vi "IO.Create.vi"(8 "error in (no error)":errorcluster, 10 "IO Control":T2 {"Signals"."Response"."Byte Order" items=["Little Endian", "Big Endian"]; "Signals"."Response"."Data Type" items=["Signed", "Unsigned", "IEEE Float"]; "Signals"."Cmd"."Byte Order" items=["Little Endian", "Big Endian"]; "Signals"."Cmd"."Data Type" items=["Signed", "Unsigned", "IEEE Float"]}, 11 "Section Ptr":T1 format="%.0x") -> (0 "error out":errorcluster, 3 "Parent Ref out":T1 format="%.0x")   [LabVIEW 2015, in "Diagnostics Addon System Explorer.lvlib"]
uses:
  Diagnostics Addon System Explorer.lvlib
  Types/IO.Export.ctl
  Types/CmdResp.Export.ctl
  Shared/Types/Signal.ctl
  <vilib>/NI Veristand/Custom Device API/Custom Device Item Ref.ctl
  Types/FG.Action.ctl
  Shared/Types/Type.ctl
  <vilib>/NI Veristand/Custom Device API/NI VeriStand - Get Item Property.vi
  <vilib>/NI Veristand/Custom Device API/Get Item Property (U32).vi
  <vilib>/NI/NI VeriStand SysDef Utilities/SysDef API/SysDef.Property.Set.vi
  <vilib>/NI/NI VeriStand SysDef Utilities/_SubVIs/SysDef.Property.Set.U32.vi
  Shared/SubVIs/Constants.vi
  Shared/Diagnostics Addon Shared.lvlib
  <vilib>/NI/NI VeriStand SysDef Utilities/System Definition Utilities.lvlib
  <vilib>/NI VeriStand/Custom Device API/Custom Device API.lvlib
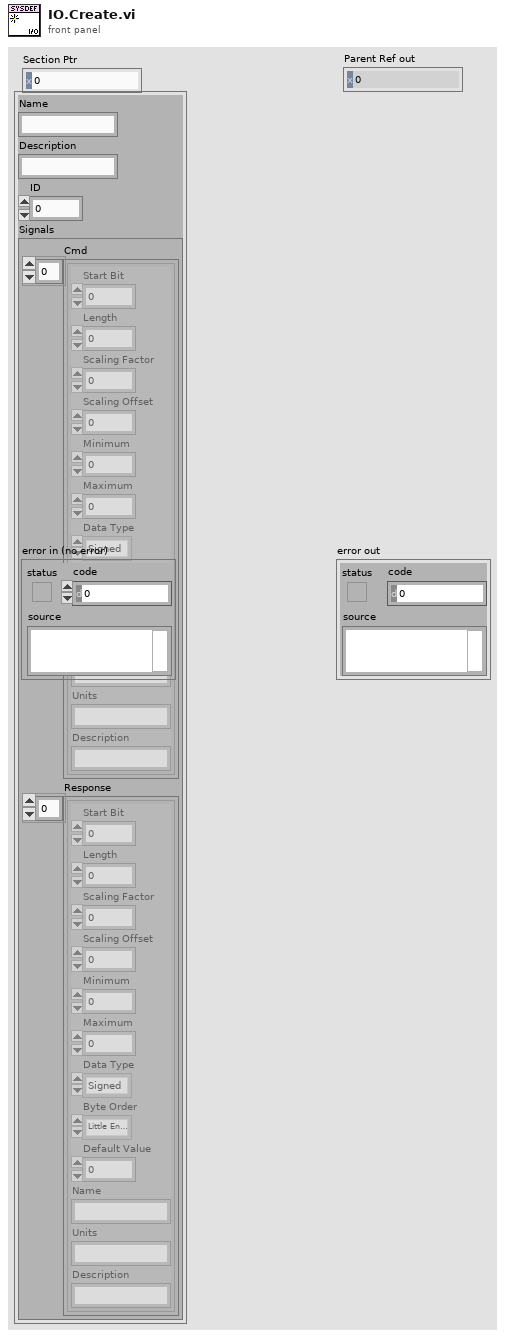
[diagram p1: front panel]
types:
  T1 = typedef "Custom Device API.lvlib/Custom Device Item Ref.ctl" = u64
  T2 = typedef "Diagnostics Addon System Explorer.lvlib/IO.Export.ctl" = cluster{"Name":string, "Description":string, "ID":u16, "Signals":T3}
  T3 = typedef "Diagnostics Addon System Explorer.lvlib/CmdResp.Export.ctl" = cluster{"Cmd":T4[], "Response":T4[]}
  T4 = typedef "Diagnostics Addon Shared.lvlib/Signal.ctl" = cluster{"Start Bit":u32, "Length":u32, "Scaling Factor":dbl, "Scaling Offset":dbl, "Minimum":dbl, "Maximum":dbl, "Data Type":u32, "Byte Order":u32, "Default Value":dbl, "Name":string, "Units":string, "Description":string}
  T5 = typedef "Diagnostics Addon Shared.lvlib/Type.ctl" = enum16{"DID", "CDID", "PID", "CPID", "Read Memory", "Write Memory", "DTC Control", "IO Cmd", "IO Resp", "Routine Start Cmd", "Routine Start Resp", "Routine Request Cmd", "Routine Request Resp", "Routine Stop Cmd", "Routine Stop Resp", "UserDefined Cmd", "UserDefined Rsp"}
  T6 = typedef "Diagnostics Addon System Explorer.lvlib/FG.Action.ctl" = enum16{"Get", "Set"}
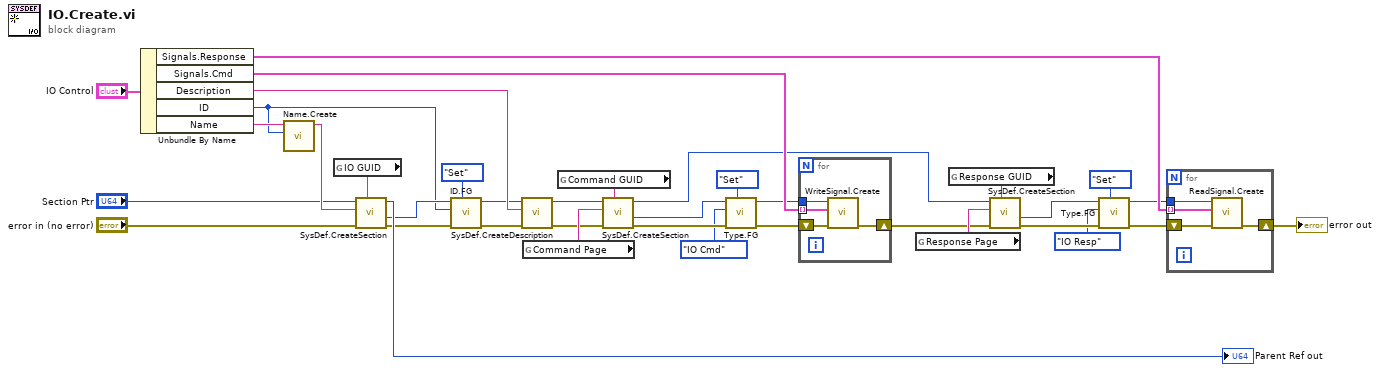
[diagram p0: block diagram]
diagram:
  n1 = Unbundle By Name("IO Control") -> ("Signals.Response"=w28:T4[], "Signals.Cmd"=w36:T4[], "Description"=w31:string, "ID"=w15:u16, "Name"=w18:string)
  n2 = call "Name.Create.vi"("PID Number"=w15, "PID Name"=w18) -> ("VS Name"=w37:string)  [unwired: 9 in]
  n3 = global read "Constants.vi" "IO GUID"() -> (w34:string)
  n4 = call <vilib>:"SysDef.CreateSection.vi"("GUID"=w34, "error in (no error)"="error in (no error)", "Name"=w37, "nodeID"="Section Ptr") -> ("error out"=w17:errorcluster, "New NodeID"=w16:u64, "nodeID out"=→"Parent Ref out":u64)  [unwired: 4 in, 1 out]
  n5 = call "ID.FG.vi"("Action"=FG.Action."Set", "error in (no error)"=w17, "ID"=w15, "Device Item Ref in"=w16) -> ("error out"=w13:errorcluster, "Device Item Ref out"=w12:T1)  [unwired: 5 in, 1 out]
  n6 = call <vilib>:"SysDef.CreateDescription.vi"("error in (no error)"=w13, "Description"=w31, "ID in"=w12) -> ("error out"=w22:errorcluster, "ID out"=w21:T1)  [unwired: 7 in]
  n7 = global read "Constants.vi" "Command Page"() -> (w27:string)
  n8 = global read "Constants.vi" "Command GUID"() -> (w26:string)
  n9 = call <vilib>:"SysDef.CreateSection.vi"("GUID"=w26, "error in (no error)"=w22, "Name"=w27, "nodeID"=w21) -> ("error out"=w10:errorcluster, "New NodeID"=w19:u64, "nodeID out"=w23:u64)  [unwired: 4 in, 1 out]
  n10 = call "Type.FG.vi"("Action"=FG.Action."Set", "error in (no error)"=w10, "Type"=Type."IO Cmd", "Device Item Ref in"=w19) -> ("error out"=w9:errorcluster, "Device Item Ref out"=w11:T1)  [unwired: 5 in, 1 out]
  n11 = for {
    shift-right: [w38] -> w20
    shift-left: w9 -> [w41]
    tunnel: w36 -> [w40] mode=indexing
    tunnel: w11 -> [w39]
    n12 = call "WriteSignal.Create.vi"("error in (no error)"=w41, "Signal Parameters"=w40, "Section Ptr"=w39) -> ("error out"=w38:errorcluster)  [unwired: 7 in, 1 out]
  }
  n13 = global read "Constants.vi" "Response Page"() -> (w24:string)
  n14 = global read "Constants.vi" "Response GUID"() -> (w25:string)
  n15 = call <vilib>:"SysDef.CreateSection.vi"("GUID"=w25, "error in (no error)"=w20, "Name"=w24, "nodeID"=w23) -> ("error out"=w6:errorcluster, "New NodeID"=w4:u64)  [unwired: 4 in, 2 out]
  n16 = call "Type.FG.vi"("Action"=FG.Action."Set", "error in (no error)"=w6, "Type"=Type."IO Resp", "Device Item Ref in"=w4) -> ("error out"=w5:errorcluster, "Device Item Ref out"=w3:T1)  [unwired: 5 in, 1 out]
  n17 = for {
    shift-right: [w44] -> w29
    shift-left: w5 -> [w45]
    tunnel: w28 -> [w43] mode=indexing
    tunnel: w3 -> [w42]
    n18 = call "ReadSignal.Create.vi"("error in (no error)"=w45, "Signal Parameters"=w43, "Section Ptr"=w42) -> ("error out"=w44:errorcluster)  [unwired: 7 in, 1 out]
  }
  "error out" <- w29
